vi "EE_EmoEngineEventHandle_Read.vi"(8 "error in (no error)":errorcluster, 11 "EmotivEpocHeadsetControls in":refnum<class "EmotivEpocHeadsetControls.lvclass">) -> (0 "error out":errorcluster, 2 "EmoEngineEventHandle":i64 caption="EmoStateHandle" format="%.0g", 3 "EmotivEpocHeadsetControls out":refnum<class "EmotivEpocHeadsetControls.lvclass">)   [LabVIEW 2016, in "Emotiv Epoc.lvlib" / "EmotivEpocHeadsetControls.lvclass"]
uses:
  EmotivEpocHeadsetControls.lvclass
  EmotivEpocHeadsetControls.lvclass/EmotivEpocHeadsetControls.ctl
panel:
  # "This VI is a part of BCI Design library, http://www.ru-bci.org \nCopyright © 2020, Sotnikov Peter, All rights reserved. License: GNU GPLv3"
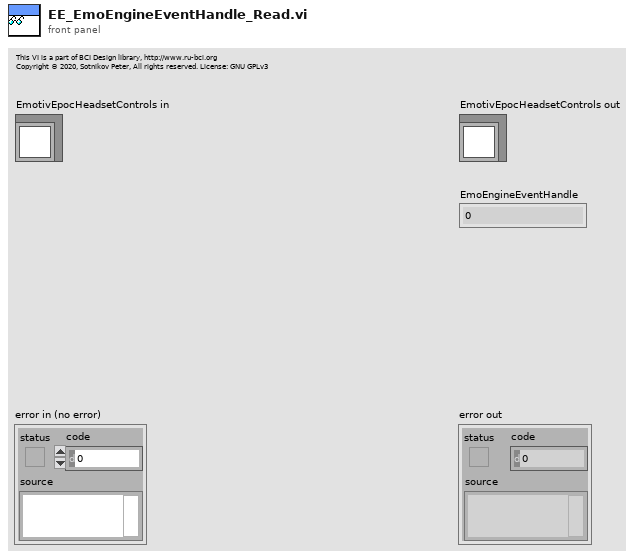
[diagram p1: front panel]
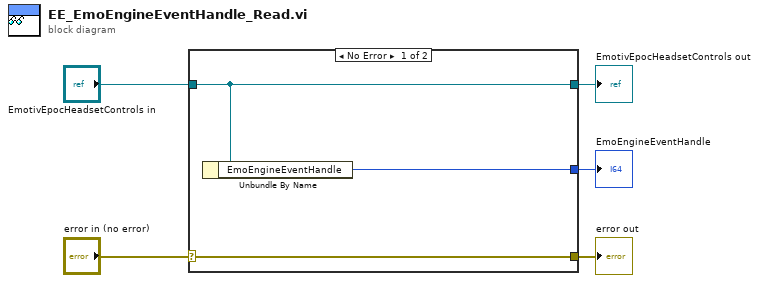
[diagram p0: block diagram]
diagram:
  n1 = case shown="No Error" "error in (no error)" {
    selector: "error in (no error)" -> [w8 w9]
    tunnel: [w8 w9] -> w4
    tunnel: [w7 w10] -> w2
    tunnel: "EmotivEpocHeadsetControls in" -> [w7 w10]
    tunnel: [w6 _] -> w1
    frame No Error {
      n2 = Unbundle By Name(w7) -> ("EmoEngineEventHandle"=w6:i64)
    }
    frame Error {
    }
  }
  "error out" <- w4
  "EmotivEpocHeadsetControls out" <- w2
  "EmoEngineEventHandle" <- w1
